vi "Write Initialization VI Properties.vi"(8 "error in (no error)":errorcluster, 10 "Initialization VI Properties":T1={"Execution"=enum."silent", "Path"={"Path"=path "", "Path Type"=enum."Absolute"}, "Type"=enum."VI", "Position"=enum."centered"}, 11 "CustomDeviceRepo in":refnum<class "CustomDeviceRepo.lvclass">) -> (0 "error out":errorcluster, 3 "CustomDeviceRepo out":refnum<class "CustomDeviceRepo.lvclass">)   [LabVIEW 2015, in "CustomDeviceRepo.lvclass"]
uses:
  CustomDeviceRepo.lvclass
  XML Controls/Initialization VI Properties.ctl
  XML Controls/Execution Types.ctl
  XML Controls/Path Cluster.ctl
  CustomDeviceRepo.lvclass/CustomDeviceRepo.ctl
  VeriStand Custom Device XML Parser.lvlib
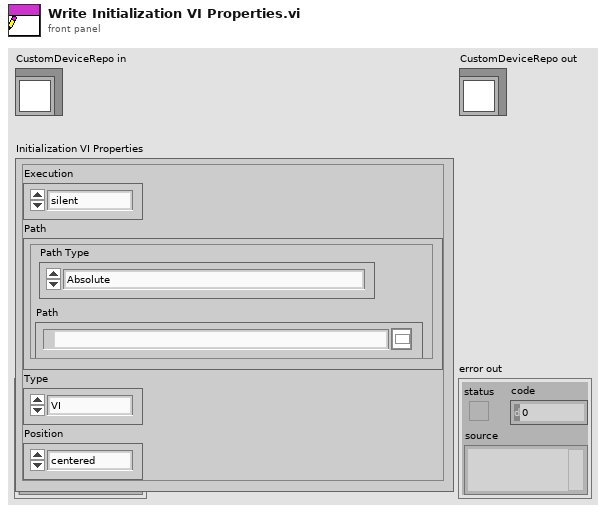
[diagram p1: front panel]
types:
  T1 = typedef "VeriStand Custom Device XML Parser.lvlib/Initialization VI Properties.ctl" = cluster{"Execution":T2, "Path":T3, "Type":enum16{"Action", "VI"}, "Position":enum16{"centered", "mouse pointer"}}
  T2 = typedef "VeriStand Custom Device XML Parser.lvlib/Execution Types.ctl" = enum16{"silent", "modal", "floating", "default"}
  T3 = typedef "VeriStand Custom Device XML Parser.lvlib/Path Cluster.ctl" = cluster{"Path":path, "Path Type":enum16{"Absolute", "To Base", "To Common Doc Dir", "To Application Data Dir"}}
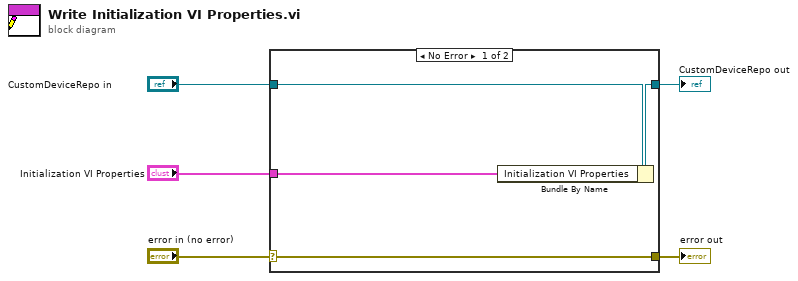
[diagram p0: block diagram]
diagram:
  n1 = case shown="No Error" "error in (no error)" {
    selector: "error in (no error)" -> [w9 w10]
    tunnel: [w9 w10] -> w4
    tunnel: [w7 w11] -> w2
    tunnel: "CustomDeviceRepo in" -> [w8 w11]
    tunnel: "Initialization VI Properties" -> [w6 _]
    frame No Error {
      n2 = Bundle By Name(cluster=w8, "Initialization VI Properties"=w6) -> (w7:refnum<class "CustomDeviceRepo.lvclass">)
    }
    frame Error {
    }
  }
  "error out" <- w4
  "CustomDeviceRepo out" <- w2
